vi "_CSMObj-Obtain.vi"(7 "Allowed Messages(Empty for all)":string[](array[string]), 8 "Error in":errorcluster caption="Error in (no error)", 11 "Requested Name":string) -> (0 "Error out":errorcluster, 3 "CSMQ out":T1={"Requested Name"="", "Module Name"="", "Mode"=enum."Stand Alone", "Queue"=refnum, "CSM-Data"=refnum, "User Event"=refnum, "Status Change Event"=refnum, "Allowed Messages"=[], "Mode-Data"=refnum, "Group Name"=""})   [LabVIEW 2014, in "Communicable State Machine.lvlib"]
uses:
  Communicable State Machine.lvlib
  _CSMObj.ctl
  Priority Queue/Priority Queue.lvclass
  Typedef/_CSM_MODE.ctl
  _CSMObj-Data.ctl
  Typedef/_CSM Status Change Event Data.ctl
  _CSMObj-ModeData.ctl
  Priority Queue/Priority Queue.lvclass/Priority Queue.ctl
  Priority Queue/Obtain Priority Queue.vi
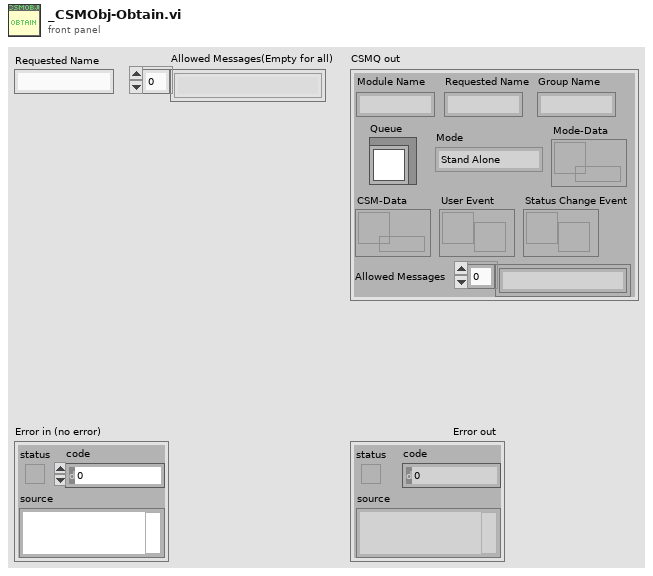
[diagram p1: front panel]
types:
  T1 = typedef "Communicable State Machine.lvlib/_CSMObj.ctl" = cluster{"Requested Name":string, "Module Name":string, "Mode":T2, "Queue":refnum<class "Priority Queue.lvclass">, "CSM-Data":refnum<data-value>, "User Event":refnum<user-event>, "Status Change Event":refnum<user-event>, "Allowed Messages":string[], "Mode-Data":refnum<data-value>, "Group Name":string}
  T2 = typedef "Communicable State Machine.lvlib/_CSM_MODE.ctl" = enum16{"Not Exist", "Stand Alone", "CSM", "Worker Agent", "Worker", "Chain", "Chain Node"}
  T3 = typedef "Communicable State Machine.lvlib/_CSMObj-ModeData.ctl" = cluster{"Share Count":i32}
  T4 = typedef "Communicable State Machine.lvlib/_CSMObj-Data.ctl" = cluster{"Locked?":bool, "RemoteMessge?":bool, "error":errorcluster}
  T5 = typedef "_CSM_NAME_REQUEST.ctl" = enum16{"Stand Alone CSM Request", "Normal CSM Request", "Agent Request", "Action Worker Request", "Chain Request", "Chain Node Request"}
  T6 = typedef "Communicable State Machine.lvlib/_CSM Status Change Event Data.ctl" = cluster{"ModuleName":string, "Status":string, "Arguments":string}
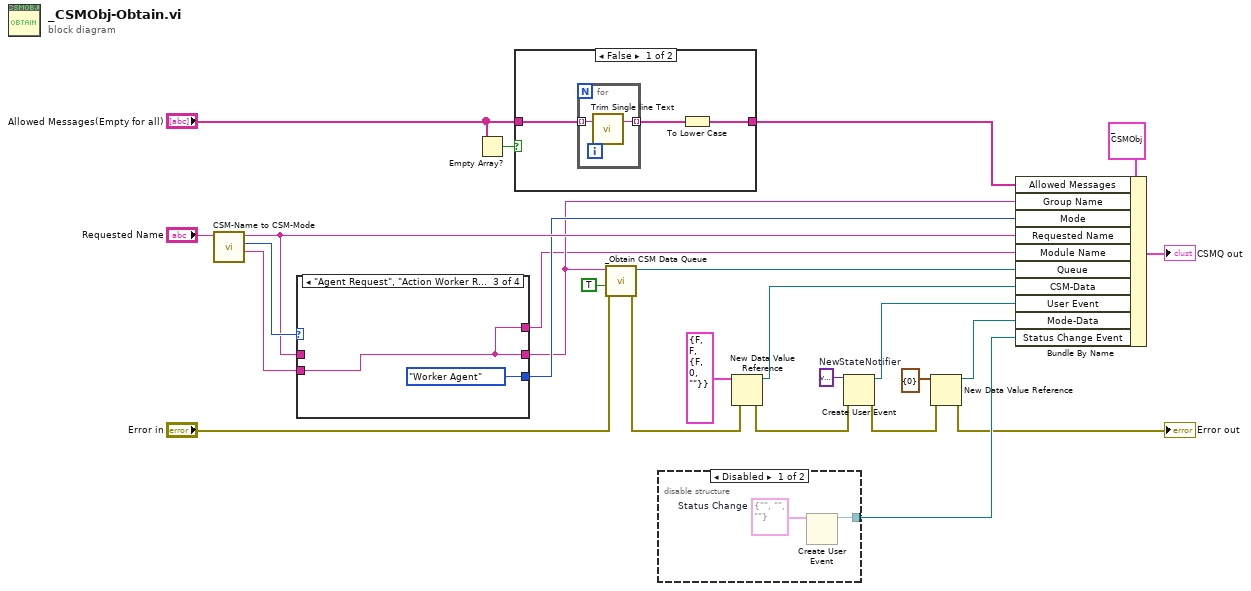
[diagram p0: block diagram]
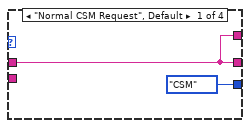
[diagram p2: hidden frame]
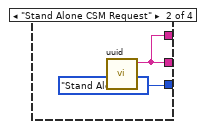
[diagram p3: hidden frame]
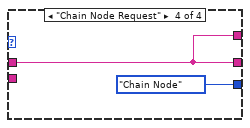
[diagram p4: hidden frame]
diagram:
  w23 = variant  # NewStateNotifier
  n1 = call "CSM-Name to CSM-Mode.vi"("String"="Requested Name") -> ("ParentCSM Name"=w12:string, "CSM Mode"=w10:T5, "Requested Name"=w9:string)  [unwired: 8 in]
  n2 = case shown="\"Agent Request\", \"Action Worker Request\"" w10 {
    tunnel: [w27 w29 w31 w33] -> w2
    tunnel: w9 -> [w27 _ _ w33]
    tunnel: w12 -> [_ _ w31 _]
    tunnel: [_CSM_MODE."CSM" ("Mode") _CSM_MODE."Stand Alone" ("Mode") _CSM_MODE."Worker Agent" ("Mode") _CSM_MODE."Chain Node" ("Mode")] -> w8
    tunnel: [w27 w29 w31 w33] -> w1
    frame "Normal CSM Request", Default {
    }
    frame "Stand Alone CSM Request" {
      n3 = call "uuid.vi"() -> ("UUID"=w29:string)  [unwired: 11 in]
    }
    frame "Agent Request", "Action Worker Request" {
    }
    frame "Chain Node Request" {
    }
  }
  n4 = Empty Array?(array="Allowed Messages(Empty for all)") -> (empty?=w13:bool)
  n5 = case shown="False" w13 {
    tunnel: [w35 w40] -> w15
    tunnel: "Allowed Messages(Empty for all)" -> [w36 w40]
    frame False {
      n6 = for {
        tunnel: [w38] -> w37 mode=indexing
        tunnel: w36 -> [w39] mode=indexing
        n7 = call "Trim Single line Text.vi"("single-line text"=w39) -> ("trimed text"=w38:string)  [unwired: 2 in]
      }
      n8 = To Lower Case(string=w37) -> (all lower case string=w35:string[])
    }
    frame True {
    }
  }
  n9 = call "_Obtain CSM Data Queue.vi"("error in (no error)"="Error in", "create if not found? (T)"=TRUE, "Name"=w2) -> ("error out"=w24:errorcluster, "Priority Queue"=w26:refnum<class "Priority Queue.lvclass">)  [unwired: 6 in, 1 out]
  n10 = disable-structure shown="Disabled" {
    disable-tunnel: [w41 _] -> w20
    frame Disabled {
      w42 = T6 {"ModuleName"="", "Status"="", "Arguments"=""}  # Status Change
      n11 = Create User Event(user event datatype=w42) -> (user event=w41:refnum<user-event>)  [unwired: 1 in, 1 out]
    }
    frame Enabled {
    }
  }
  n12 = New Data Value Reference(data value=T4 {"Locked?"=FALSE, "RemoteMessge?"=FALSE, "error"={"status"=FALSE, "code"=0, "source"=""}} ("CSMObj-Data"), error in=w24) -> (data value reference=w25:refnum<data-value>, error out=w22:errorcluster)
  n13 = Create User Event(user event datatype=w23, error in=w22) -> (user event=w21:refnum<user-event>, error out=w4:errorcluster)
  n14 = New Data Value Reference(data value=T3 {"Share Count"=0} ("CSMObj-Data"), error in=w4) -> (data value reference=w5:refnum<data-value>, error out=→"Error out":errorcluster)
  n15 = Bundle By Name(cluster=T1 {"Requested Name"="", "Module Name"="", "Mode"=enum."Stand Alone", "Queue"=refnum, "CSM-Data"=refnum, "User Event"=refnum, "Status Change Event"=refnum, "Allowed Messages"=[], "Mode-Data"=refnum, "Group Name"=""} ("CSMQ in"), "Allowed Messages"=w15, "Group Name"=w2, "Mode"=w8, "Requested Name"=w9, "Module Name"=w1, "Queue"=w26, "CSM-Data"=w25, "User Event"=w21, "Mode-Data"=w5, "Status Change Event"=w20) -> (→"CSMQ out":T1)
